vi "IR align.vi"(2 "Banchmark in":T2={"DC estimate (V)2"=1.2526850823671394, "DC estimate (V)1"=2.565470433392377}, 3 "IR in":T1) -> (0 "x*y":dbl[](array[numeric]), 1 "x > y?":bool)   [LabVIEW 2019]
uses:
  alignment benchmark.ctl
  distance measure/IR/IR out.ctl
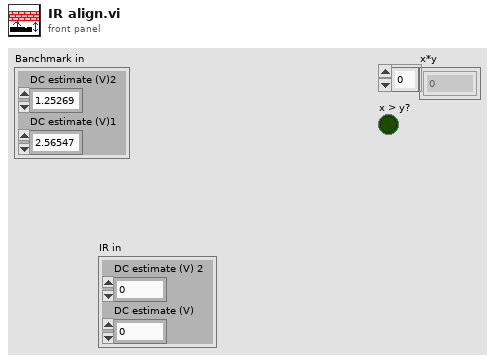
[diagram p1: front panel]
types:
  T1 = typedef "IR out.ctl" = cluster{"DC estimate (V) 2":dbl, "DC estimate (V)":dbl}
  T2 = typedef "alignment benchmark.ctl" = cluster{"DC estimate (V)2":dbl, "DC estimate (V)1":dbl}
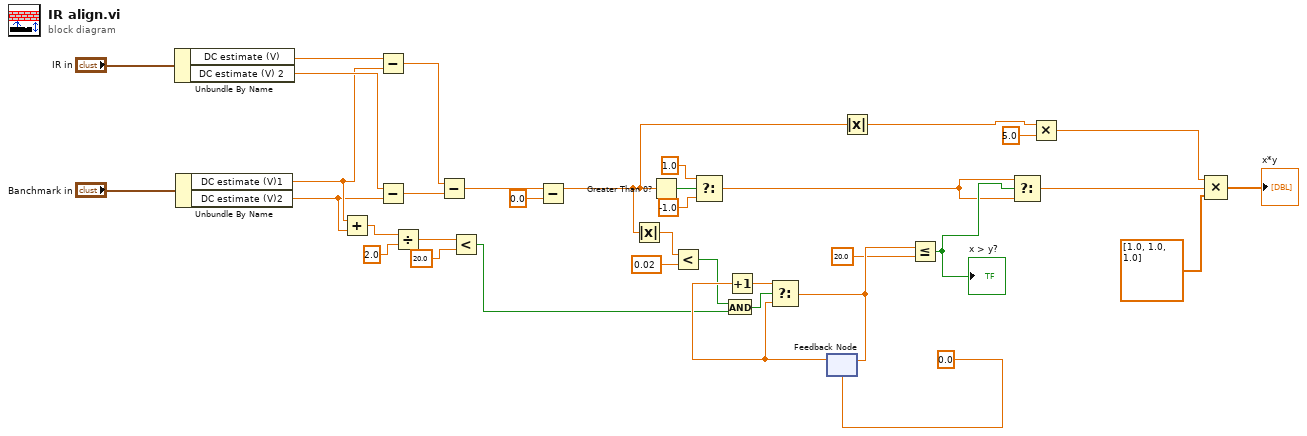
[diagram p0: block diagram]
diagram:
  n1 = Unbundle By Name("IR in") -> ("DC estimate (V)"=w34:dbl, "DC estimate (V) 2"=w33:dbl)
  n2 = Unbundle By Name("Banchmark in") -> ("DC estimate (V)1"=w7:dbl, "DC estimate (V)2"=w6:dbl)
  n3 = Add(x=w7, y=w6) -> (x+y=w5:dbl)
  n4 = Subtract(x=w34, y=w7) -> (x-y=w31:dbl)
  n5 = Subtract(x=w33, y=w6) -> (x-y=w32:dbl)
  n6 = Divide(x=w5, y=2.0) -> (x/y=w3:dbl)
  n7 = Subtract(x=w31, y=w32) -> (x-y=w20:dbl)
  n8 = Less?(x=w3, y=20.0) -> (x < y?=w1:bool)
  n9 = Subtract(x=w20, y=0.0) -> (x-y=w12:dbl)
  n10 = Absolute Value(x=w12) -> (abs(x)=w19:dbl)
  n11 = Greater Than 0?(x=w12) -> (x > 0?=w30:bool)
  n12 = Less?(x=w19, y=0.02) -> (x < y?=w8:bool)
  n13 = Select(t=1.0 ("f"), s=w30, f=-1.0) -> (s? t:f=w10:dbl)
  n14 = And(x=w8, y=w1) -> (x .and. y?=w9:bool)
  n15 = feedback #1(0.0 ("f")) -> (w16:dbl)
  n16 = Increment(x=w16) -> (x+1=w17:dbl)
  n17 = Select(t=w17, s=w9, f=w16) -> (s? t:f=w15:dbl)
  n18 = feedback-in #1(w15) -> ()
  n19 = Absolute Value(x=w12) -> (abs(x)=w21:dbl)
  n20 = Less Or Equal?(x=w15, y=20.0) -> (x <= y?=w13:bool)
  "x > y?" <- w13
  n21 = Select(t=w10, s=w13, f=w10) -> (s? t:f=w23:dbl)
  n22 = Multiply(x=w21, y=5.0) -> (x*y=w25:dbl)
  n23 = Compound Arithmetic op=MULTIPLY(w25, w23, dbl[] [1.0, 1.0, 1.0]) -> (→"x*y":dbl[])
